vi "Test1.vi"() -> ()   [LabVIEW 2017]
panel:
  out "x*y":dbl
  in  "Numeric":dbl format="%#_13g"
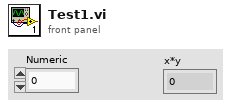
[diagram p1: front panel]
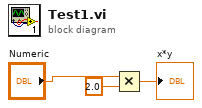
[diagram p0: block diagram]
diagram:
  n1 = Multiply(x="Numeric", y=2.0) -> (x*y=→"x*y":dbl)
